vi "DataStream_Write Data.vi"(6 "Header Array":string[](array[string]), 8 "Error":errorcluster, 9 "Value Array":dbl[](array[numeric]), 10 "Time Stamp Array":dbl[](array[numeric]), 11 "Time Stamp For ALL":dbl) -> (0 "Error Out":errorcluster, 3 "Data Sent Out":T1)   [LabVIEW 2023]
uses:
  TypeDefs/Cluster_DataStream RT Data Set.ctl
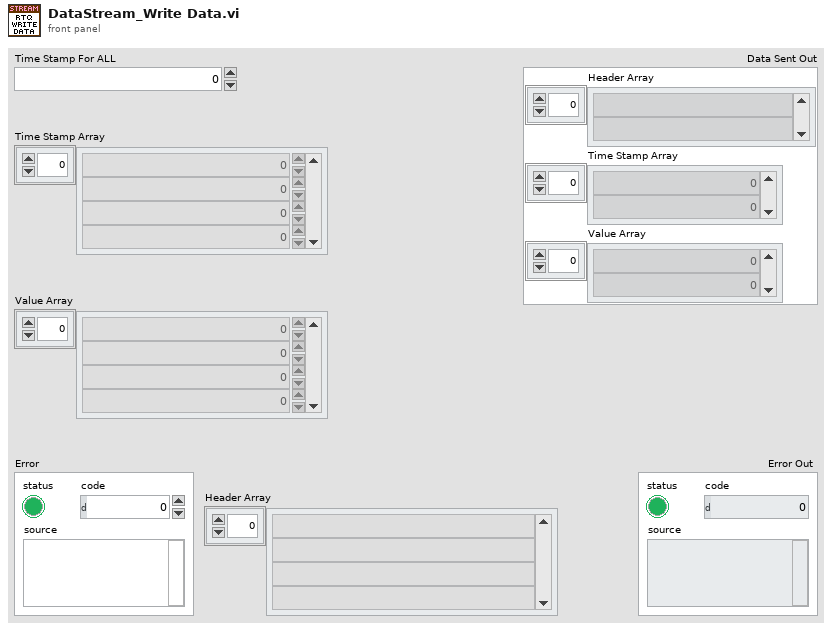
[diagram p1: front panel]
types:
  T1 = typedef "Cluster_DataStream RT Data Set.ctl" = cluster{"Header Array":string[], "Time Stamp Array":dbl[], "Value Array":dbl[]}
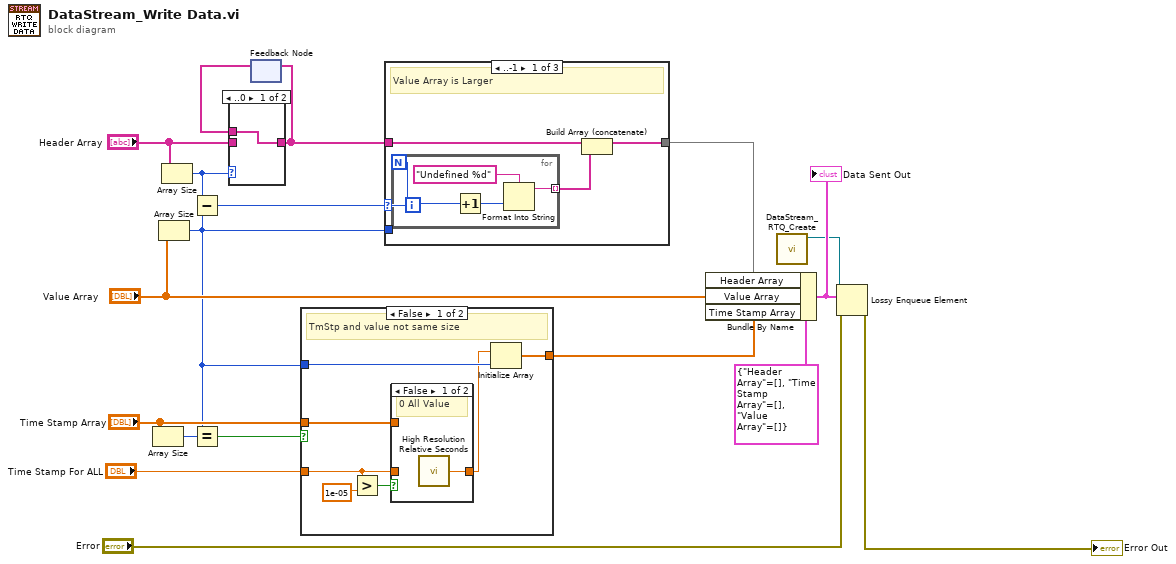
[diagram p0: block diagram]
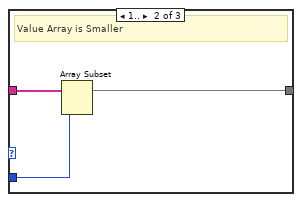
[diagram p2: hidden frame]
diagram:
  n1 = Array Size(array="Time Stamp Array") -> (size(s)=w11:i32)
  n2 = Array Size(array="Value Array") -> (size(s)=w5:i32)
  n3 = Array Size(array="Header Array") -> (size(s)=w13:i32)
  n4 = Subtract(x=w13, y=w5) -> (x-y=w12:i32)
  n5 = Equal?(x=w5, y=w11) -> (x = y?=w9:bool)
  n6 = feedback #1() -> (w14:string[])  [unwired: 1 in]
  n7 = case shown="..0" w13 {
    tunnel: "Header Array" -> [_ w20]
    tunnel: [w19 w20] -> w4
    tunnel: w14 -> [w19 _]
    frame ..0 {
    }
    frame 1.. {
    }
  }
  n8 = feedback-in #1(w4) -> ()
  n9 = case shown="False" w9 {
    tunnel: "Time Stamp Array" -> [w25 w30]
    tunnel: [w23 w30] -> w7
    tunnel: "Time Stamp For ALL" -> [w22 _]
    tunnel: w5 -> [w24 _]
    frame False {
      # "TmStp and value not same size"
      n10 = Greater?(x=w22, y=1e-05) -> (0:w26:bool)
      n11 = case shown="False" w26 {
        tunnel: w25 -> [_ _]
        tunnel: w22 -> [_ w29]
        tunnel: [w28 w29] -> w21
        frame False {
          # "0 All Value"
          n12 = call <vilib>:"High Resolution Relative Seconds.vi"() -> ("relative seconds"=w28:dbl)
        }
        frame True {
          # "Valid All Value"
        }
      }
      n13 = Initialize Array(w21, w24) -> (w23:dbl[])
    }
    frame True {
      # "Time Stamp and Value Array same size"
    }
  }
  n14 = case shown="..-1" w12 {
    selector: w12 -> [w34 _ _]
    tunnel: w4 -> [w32 w41 w42]
    tunnel: [w31 w39 w42] -> w3
    tunnel: w5 -> [_ w40 _]
    frame ..-1 {
      # "Value Array is Larger"
      n15 = for {
        N: w34 -> [_]
        tunnel: [w35] -> w33 mode=indexing
        i -> [w37]
        n16 = Increment(x=w37) -> (x+1=w36:i32)
        n17 = Format Into String(format string="Undefined %d", w36) -> (resulting string=w35:string)  [unwired: 2 in, 1 out]
      }
      n18 = Build Array (concatenate)(w32, w33) -> (w31:string[])
    }
    frame 1.. {
      # "Value Array is Smaller"
      n19 = Array Subset(array=w41, length=w40) -> (w39:string[])  [unwired: 1 in]
    }
    frame 0 {
      # "Equal in Size"
    }
  }
  n20 = Bundle By Name(cluster=T1 {"Header Array"=[], "Time Stamp Array"=[], "Value Array"=[]} ("element"), "Header Array"=w3, "Value Array"="Value Array", "Time Stamp Array"=w7) -> (w16:T1)
  "Data Sent Out" <- w16
  n21 = call "DataStream_RTQ_Create.vi"() -> ("RTQ"=w1:refnum<queue>)  [unwired: 11 in]
  n22 = Lossy Enqueue Element(queue=w1, element=w16, error in (no error)="Error") -> (error out=→"Error Out":errorcluster)  [unwired: 3 out]
